vi "Configure All By Config.vi"(8 "error in":errorcluster, 11 "ActorMeter in":refnum<class "ActorMeter.lvclass">) -> (0 "error out":errorcluster, 3 "ActorMeter out":refnum<class "ActorMeter.lvclass">)   [LabVIEW 2014, in "ActorMeter.lvclass"]
uses:
  ActorMeter.lvclass
  SimpleExperimentService/SimpleExperimentService.lvclass
  <vilib>/ActorFramework/Actor/Actor.lvclass/Actor.ctl
  <vilib>/ActorFramework/Message Enqueuer/Message Enqueuer.lvclass/Message Enqueuer.ctl
  ActorMeter.lvclass/ActorMeter.ctl
  ExperimentService/ExperimentService.lvclass/ExperimentService.ctl
  StorageService/StorageService.lvclass
  Model/Data/MessageToSend.ctl
  <vilib>/ActorFramework/Message Enqueuer/Message Enqueuer.lvclass
  <vilib>/ActorFramework/Message/Message.lvclass
  ExperimentService/ExperimentService Messages/Set Next Parameter Msg/Set Next Parameter Msg.lvclass
  <vilib>/Utility/sysdir.llb/System Directory Type.ctl
  ExperimentService/ExperimentService Messages/Write StorageService Msg/Write StorageService Msg.lvclass/Write StorageService Msg.ctl
  Model/ReplayData Msg/ReplayData Msg.lvclass
  Hardware/ParameterDevice/ParameterDevice Messages/Get Parameter Msg/Get Parameter Msg.lvclass
  Interfaces/Observable Actor/Read Data Msg/Read Data Msg.lvclass
  <vilib>/ActorFramework/Message Enqueuer/Message Priority.ctl
  StorageService/StorageService Messages/Register Msg/Register Msg.lvclass/Register Msg.ctl
  StorageService/StorageService Messages/Notify All Objects Msg/Notify All Objects Msg.lvclass
  Interfaces/Observable Actor/Observable Actor Messages/Add On Event Message Msg/Add On Event Message Msg.lvclass/Add On Event Message Msg.ctl
  <vilib>/ActorFramework/Message Enqueuer/Init from Existing Queue.vi
  <vilib>/ActorFramework/Message Enqueuer/Enqueue.vi
  <vilib>/ActorFramework/Message Priority Queue/Priority Enqueue.vi
  ExperimentService/ExperimentService Messages/Write StorageService Msg/Write StorageService Msg.lvclass
  Extractor/AbstractExtractor/AbstractExtractor.lvclass
  StorageService/StorageService Messages/Register Msg/Register Msg.lvclass
  Interfaces/Observable Actor/Observable Actor Messages/Add On Event Message Msg/Add On Event Message Msg.lvclass
  <vilib>/ActorFramework/Actor/Actor.lvclass
  ExperimentService/ExperimentService.lvclass
  Interfaces/Observable Actor/Observable Actor.lvclass
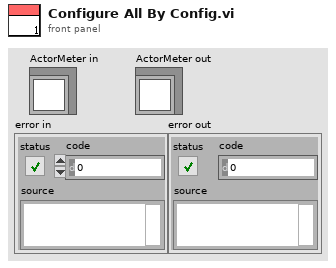
[diagram p1: front panel]
types:
  T1 = typedef "MessageToSend.ctl" = cluster{"Enqueuer":refnum<class "Message Enqueuer.lvclass">, "Message":refnum<class "Message.lvclass">}
  T2 = cluster{"Enqueuer":refnum<class "Message Enqueuer.lvclass">, "Message":refnum<class "ReplayData Msg.lvclass">}
  T3 = typedef "Actor Framework.lvlib/Message Enqueuer.lvclass/Message Priority.ctl" = enum16{"Low", "Normal", "High"}
  T4 = typedef "System Directory Type.ctl" = i32
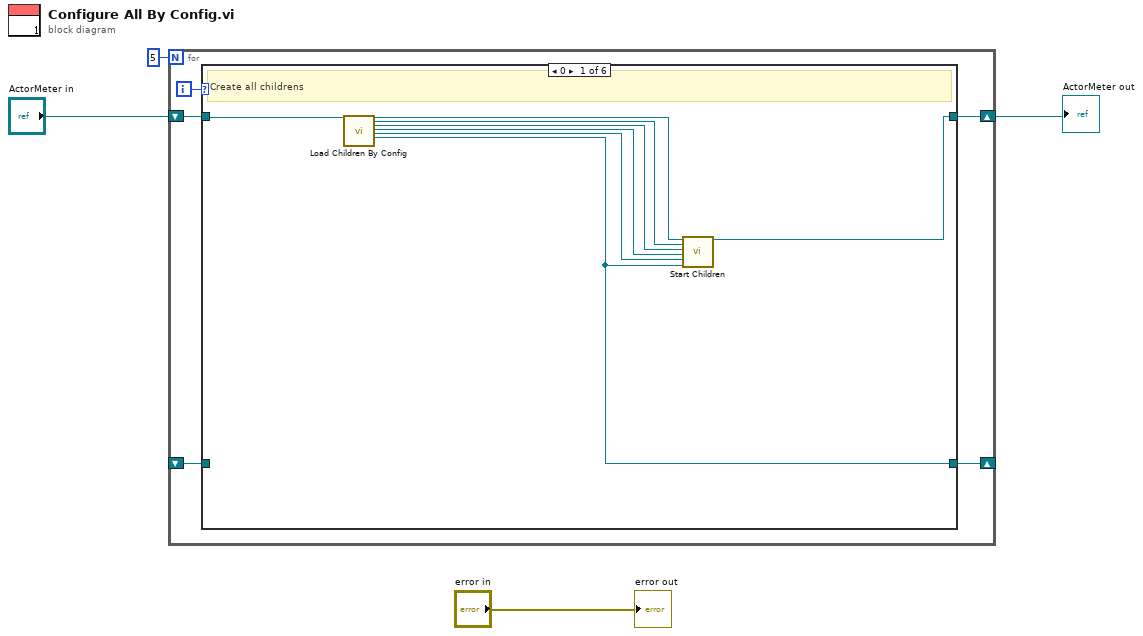
[diagram p0: block diagram]
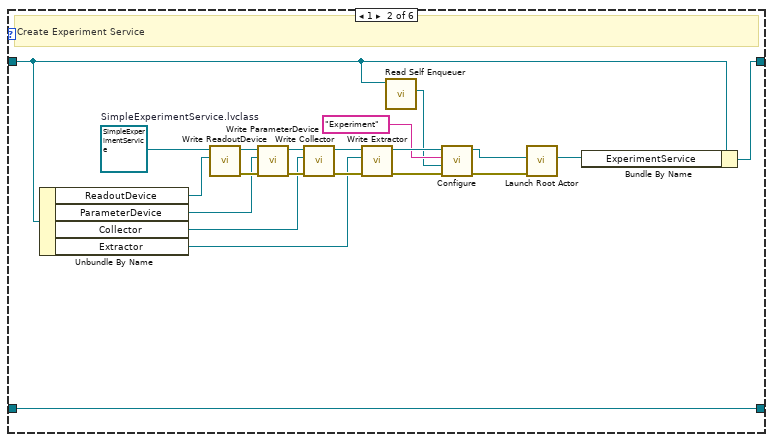
[diagram p2: hidden frame]
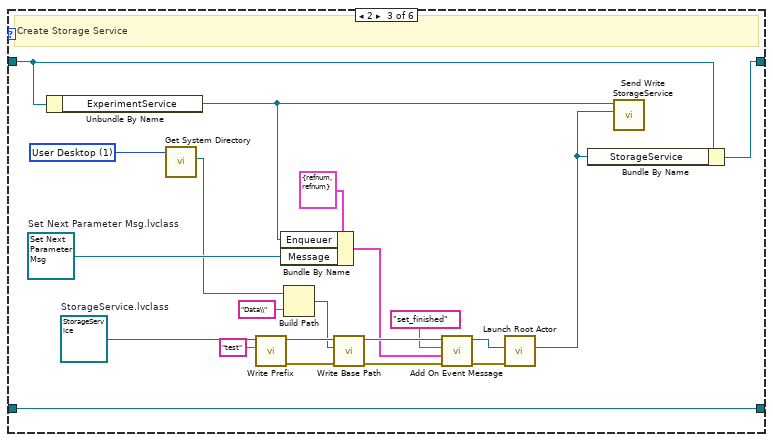
[diagram p3: hidden frame]
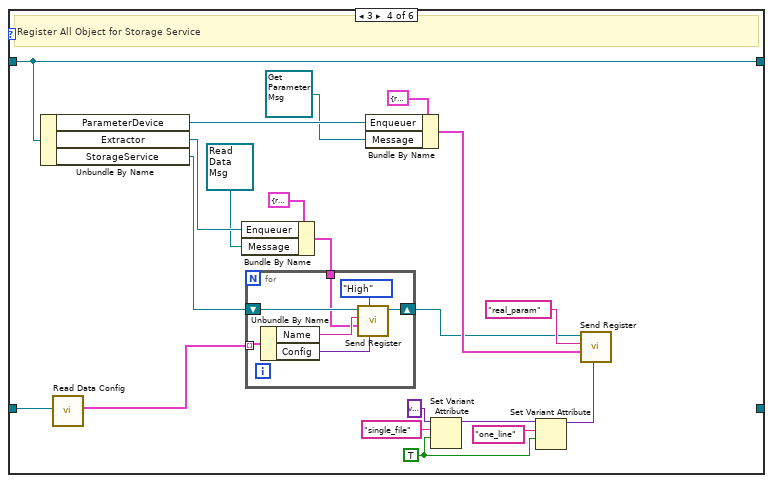
[diagram p4: hidden frame]
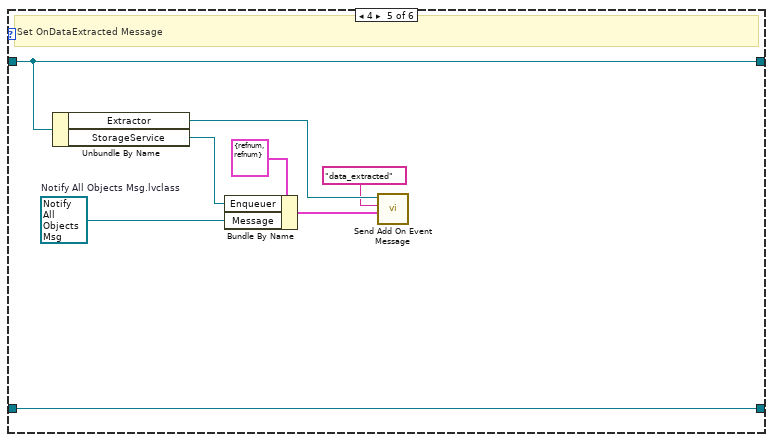
[diagram p5: hidden frame]
diagram:
  n1 = for {
    N: 5 -> [_]
    shift-right: [w8] -> w2
    shift-left: "ActorMeter in" -> [w9]
    shift-right: [w6] -> _
    shift-left: _ -> [w5]
    i -> [w7]
    n2 = case shown="0" w7 {
      tunnel: w9 -> [w16 w19 w53 w79 w94 w95]
      tunnel: [w17 w30 w52 w79 w94 w95] -> w8
      tunnel: [w10 w29 w39 _ w87 _] -> w6
      tunnel: w5 -> [_ w29 w39 w64 w87 _]
      frame 0 {
        # "Create all childrens"
        n3 = call "Load Children By Config.vi"("ActorMeter in"=w16) -> ("ActorMeter out"=w15:refnum<class "ActorMeter.lvclass">, "ParameterDevice.lvclass"=w14:refnum<class "ParameterDevice.lvclass">, "ReadoutDevice.lvclass"=w13:refnum<class "ReadoutDevice.lvclass">, "AbstractProcessor.lvclass"=w12:refnum<class "AbstractProcessor.lvclass">, "AbstractCollector.lvclass"=w11:refnum<class "AbstractCollector.lvclass">, "AbstractExtractor.lvclass"=w10:refnum<class "AbstractExtractor.lvclass">)  [unwired: 20 in, 1 out]
        n4 = call "Start Children.vi"("ActorMeter in"=w15, "ParameterDevice.lvclass"=w14, "ReadoutDevice.lvclass"=w13, "AbstractProcessor.lvclass"=w12, "AbstractCollector.lvclass"=w11, "AbstractExtractor.lvclass"=w10) -> ("ActorMeter out"=w17:refnum<class "ActorMeter.lvclass">)  [unwired: 13 in]
      }
      frame 1 {
        w28 = refnum<class "SimpleExperimentService.lvclass"> refnum  # SimpleExperimentService.lvclass
        # "Create Experiment Service"
        n5 = Unbundle By Name(w19) -> ("ReadoutDevice"=w34:refnum<class "Message Enqueuer.lvclass">, "ParameterDevice"=w35:refnum<class "Message Enqueuer.lvclass">, "Collector"=w33:refnum<class "Message Enqueuer.lvclass">, "Extractor"=w25:refnum<class "Message Enqueuer.lvclass">)
        n6 = call "Write ReadoutDevice.vi"("ReadoutDevice"=w34, "ExperimentService in"=w28) -> ("error out"=w36:errorcluster, "ExperimentService out"=w31:refnum<class "SimpleExperimentService.lvclass">)  [unwired: 8 in]
        n7 = call "Write ParameterDevice.vi"("error in (no error)"=w36, "Parameter Device"=w35, "ExperimentService in"=w31) -> ("error out"=w37:errorcluster, "ExperimentService out"=w32:refnum<class "SimpleExperimentService.lvclass">)  [unwired: 7 in]
        n8 = call "Write Collector.vi"("error in (no error)"=w37, "Collector"=w33, "ExperimentService in"=w32) -> ("error out"=w26:errorcluster, "ExperimentService out"=w27:refnum<class "SimpleExperimentService.lvclass">)  [unwired: 7 in]
        n9 = call-dynamic "Write Extractor.vi"("error in (no error)"=w26, "Extractor"=w25, "ExperimentService in"=w27) -> ("error out"=w23:errorcluster, "ExperimentService out"=w24:refnum<class "SimpleExperimentService.lvclass">)  [unwired: 7 in]
        n10 = call <vilib>:"Read Self Enqueuer.vi"("Actor"=w19) -> ("Self Enqueuer"=w18:refnum<class "Message Enqueuer.lvclass">)  [unwired: 10 in]
        n11 = call-dynamic "Configure.vi"("error in (no error)"=w23, "ActorMeter Enqueuer"=w18, "Name"="Experiment", "Viewable Actor in"=w24) -> ("error out"=w21:errorcluster, "Viewable Actor out"=w22:refnum<class "SimpleExperimentService.lvclass">)  [unwired: 6 in]
        n12 = call <vilib>:"Launch Root Actor.vi"("error in (no error)"=w21, "Actor"=w22) -> ("Actor's Enqueuer"=w38:refnum<class "Message Enqueuer.lvclass">)  [unwired: 8 in, 1 out]
        n13 = Bundle By Name(cluster=w19, "ExperimentService"=w38) -> (w30:refnum<class "ActorMeter.lvclass">)
      }
      frame 2 {
        w41 = T4 1 items=["User Home"=0, "User Desktop"=1, "User Documents"=2, "User Application Data"=3, "User Preferences"=4, "User Temporary"=5, "Public Documents"=6, "Public Application Data"=7, "Public Preferences"=8, "Public Cache"=13, "System Core Libraries"=9, "System Installed Libraries"=10, "Application Files"=11, "Boot Volume Root"=12] ("system directory type")
        w59 = refnum<class "Set Next Parameter Msg.lvclass"> refnum  # Set Next Parameter Msg.lvclass
        w56 = refnum<class "StorageService.lvclass"> refnum  # StorageService.lvclass
        # "Create Storage Service"
        n14 = Unbundle By Name(w53) -> ("ExperimentService"=w51:refnum<class "Message Enqueuer.lvclass">)
        n15 = call <vilib>:"Get System Directory.vi"("system directory type"=w41) -> ("system directory"=w40:path)  [unwired: 10 in]
        n16 = call-dynamic "Write Prefix.vi"("Prefix"="test", "StorageService in"=w56) -> ("error out"=w54:errorcluster, "StorageService out"=w55:refnum<class "StorageService.lvclass">)  [unwired: 8 in]
        n17 = Bundle By Name(cluster=T1 {"Enqueuer"=refnum, "Message"=refnum} ("Message To Send"), "Enqueuer"=w51, "Message"=w59) -> (w43:T1)
        n18 = Build Path(base path=w40, name or relative path="Data\\") -> (appended path=w48:path)
        n19 = call-dynamic "Write Base Path.vi"("error in (no error)"=w54, "Base Path"=w48, "StorageService in"=w55) -> ("error out"=w45:errorcluster, "StorageService out"=w47:refnum<class "StorageService.lvclass">)  [unwired: 7 in]
        n20 = call "Add On Event Message.vi"("error in (no error)"=w45, "Message To Send"=w43, "Event"="set_finished", "Observable Actor in"=w47) -> ("error out"=w44:errorcluster, "Observable Actor out"=w46:refnum<class "StorageService.lvclass">)  [unwired: 6 in]
        n21 = call <vilib>:"Launch Root Actor.vi"("error in (no error)"=w44, "Actor"=w46) -> ("Actor's Enqueuer"=w50:refnum<class "Message Enqueuer.lvclass">)  [unwired: 8 in, 1 out]
        n22 = Bundle By Name(cluster=w53, "StorageService"=w50) -> (w52:refnum<class "ActorMeter.lvclass">)
        n23 = call "Send Write StorageService.vi"("StorageService"=w50, "Message Enqueuer"=w51) -> ()  [unwired: 8 in, 2 out]
      }
      frame 3 {
        w67 = TRUE ("Save to single file")
        # "Register All Object for Storage Service"
        n24 = Unbundle By Name(w79) -> ("ParameterDevice"=w77:refnum<class "Message Enqueuer.lvclass">, "Extractor"=w72:refnum<class "Message Enqueuer.lvclass">, "StorageService"=w61:refnum<class "Message Enqueuer.lvclass">)
        n25 = call-dynamic "Read Data Config.vi"("Observable Actor in"=w64) -> ("Extracted Data Info"=w63:cluster{"Name":string, "Config":variant}[])  [unwired: 8 in, 2 out]
        n26 = Bundle By Name(cluster=T2 {"Enqueuer"=refnum, "Message"=refnum} ("GetData Message"), "Enqueuer"=w72, "Message"=refnum<class "Read Data Msg.lvclass"> refnum ("Observable Actor.lvlib:Read Data Msg.lvclass")) -> (w62:T2)
        n27 = for {
          tunnel: w63 -> [w86] mode=indexing
          tunnel: w62 -> [w81]
          shift-right: [w84] -> w60
          shift-left: w61 -> [w85]
          n28 = Unbundle By Name(w86) -> ("Name"=w83:string, "Config"=w82:variant)
          n29 = call "Send Register.vi"("Save Parameters"=w82, "Message Priority (Normal)"=Message_Priority."High", "GetData Message"=w81, "Name"=w83, "Message Enqueuer"=w85) -> ("Message Enqueuer out"=w84:refnum<class "Message Enqueuer.lvclass">)  [unwired: 5 in, 1 out]
        }
        n30 = Bundle By Name(cluster=T2 {"Enqueuer"=refnum, "Message"=refnum} ("GetData Message"), "Enqueuer"=w77, "Message"=refnum<class "Get Parameter Msg.lvclass"> refnum ("Get Parameter Msg.lvclass")) -> (w74:T2)
        n31 = Set Variant Attribute(Variant=variant ("variant"), name="single_file", value=w67) -> (Variant out=w69:variant)  [unwired: 1 in, 2 out]
        n32 = Set Variant Attribute(Variant=w69, name="one_line", value=w67) -> (Variant out=w66:variant)  [unwired: 1 in, 2 out]
        n33 = call "Send Register.vi"("Save Parameters"=w66, "GetData Message"=w74, "Name"="real_param", "Message Enqueuer"=w60) -> ()  [unwired: 6 in, 2 out]
      }
      frame 4 {
        w91 = refnum<class "Notify All Objects Msg.lvclass"> refnum  # Notify All Objects Msg.lvclass
        # "Set OnDataExtracted Message"
        n34 = Unbundle By Name(w94) -> ("Extractor"=w90:refnum<class "Message Enqueuer.lvclass">, "StorageService"=w92:refnum<class "Message Enqueuer.lvclass">)
        n35 = Bundle By Name(cluster=T1 {"Enqueuer"=refnum, "Message"=refnum} ("Message To Send"), "Enqueuer"=w92, "Message"=w91) -> (w89:T1)
        n36 = call "Send Add On Event Message.vi"("Message To Send"=w89, "Event"="data_extracted", "Message Enqueuer"=w90) -> ()  [unwired: 7 in, 2 out]
      }
      frame Default {
      }
    }
  }
  "ActorMeter out" <- w2
  "error out" <- "error in"
